vi "Activate-lasing.vi"(8 "error in (no error)":errorcluster, 11 "Object ref in":T1) -> (0 "error out":errorcluster, 1 "Succes?":bool, 3 "Object ref out":T1)   [LabVIEW 2013, in "SLMControl.lvlib" / "SC-Main.lvclass"]
doc: "Attempts to obtain a reference to the SM1000 .NET dll libraries and to establish a TCP connection."
uses:
  SC-Main.lvclass
  Object-reference.ctl
  UI/Control-names.ctl
  Vision-actions.ctl
  SC-Main.lvclass/SC-Main.ctl
  Read Lasing control.vi
  Read UI.vi
  UI/Set-control-string.vi
  SM1000/SM1000.lvclass
  UI/SC-UI.lvclass
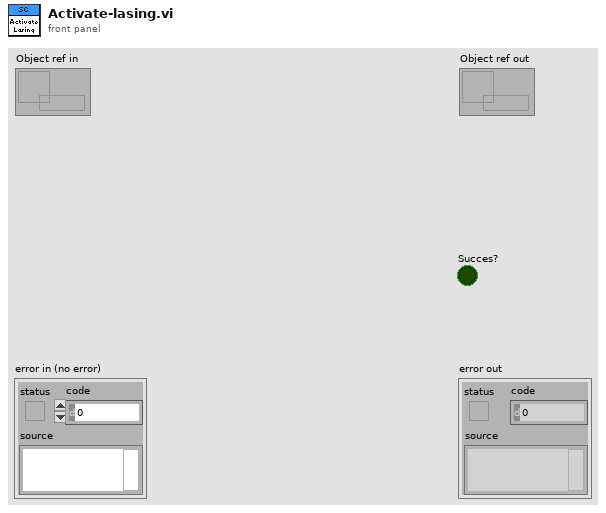
[diagram p1: front panel]
types:
  T1 = typedef "SLMControl.lvlib/SC-Main.lvclass/Object-reference.ctl" = refnum<data-value>
  T2 = typedef "SLMControl.lvlib/SC-Main.lvclass/Vision-actions.ctl" = enum16{"Activate", "Start", "Repeat", "Stop", "Exit"}
  T3 = typedef "SLMControl.lvlib/SC-UI.lvclass/Control-names.ctl" = enum16{"Com-in", "Com-out", "Help", "Status", "Load configuration", "Save configuration", "Load lasing files", "Load deposition files", "Clear", "Files", "Activate", "Execute", "Abort", "Options", "Current layer", "Current iteration", "Last elapsed time", "Deposition status", "Lasing job", "Status LEDs", "Exiting led", "Initialized led", "Files loaded led", "Activated led", "Executing led", "Deposition led", "Lasing job led", "Lasing led"}
  T4 = typedef "SLMControl.lvlib/SM1000.lvclass/Object-reference.ctl" = refnum<data-value>
  T5 = typedef "SLMControl.lvlib/SC-UI.lvclass/Panes-reference.ctl" = refnum<data-value>
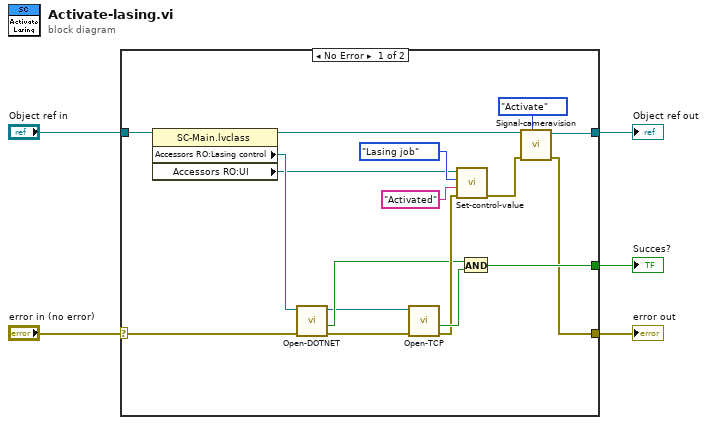
[diagram p0: block diagram]
diagram:
  n1 = case shown="No Error" "error in (no error)" {
    selector: "error in (no error)" -> [w21 w24]
    tunnel: [w6 w24] -> w4
    tunnel: [w8 w23] -> w2
    tunnel: "Object ref in" -> [w22 w23]
    tunnel: [w18 _] -> w1
    frame No Error {
      n2 = property class="SC-Main.lvclass"(reference=w22) -> (reference out=w9:T1, "Accessors RO:Lasing control"=w20:T4, "Accessors RO:UI"=w15:T5)  [unwired: 1 in, 1 out]
      n3 = call "Open-DOTNET.vi"("error in (no error)"=w21, "SM1000-control in"=w20) -> ("error out"=w12:errorcluster, "Succes?"=w13:bool, "SM1000-control out"=w11:T4)  [unwired: 7 in]
      n4 = call "Open-TCP.vi"("error in (no error)"=w12, "SM1000-control in"=w11) -> ("error out"=w14:errorcluster, "Succes?"=w19:bool)  [unwired: 7 in, 1 out]
      n5 = call-poly "Set-control-value.vi"("error in (no error)"=w14, "Value"="Activated", "Control name"=Control-names."Lasing job", "Panes in"=w15) -> ("error out"=w7:errorcluster)  [unwired: 6 in, 1 out]
      n6 = And(x=w13, y=w19) -> (x .and. y?=w18:bool)
      n7 = call "Signal-cameravision.vi"("Vision action"=Vision-actions."Activate", "error in (no error)"=w7, "Object ref in"=w9) -> ("error out"=w6:errorcluster, "Object ref out"=w8:T1)  [unwired: 7 in]
    }
    frame Error {
    }
  }
  "error out" <- w4
  "Object ref out" <- w2
  "Succes?" <- w1
